vi "Resampling app.vi"() -> ()   [LabVIEW 2018]
panel:
  in  "file path (use dialog)":path
  out "error out":errorcluster
  in  "error in":errorcluster
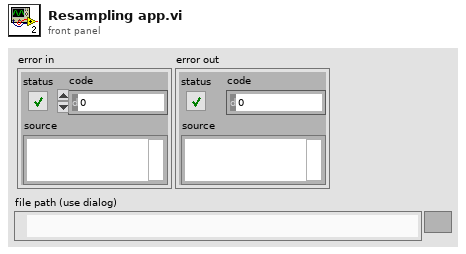
[diagram p1: front panel]
types:
  T1 = enum16{"big-endian, network order", "native, host order", "little-endian"}
  T2 = enum16{"open", "replace", "create", "open or create", "replace or create", "replace or create with confirmation"}
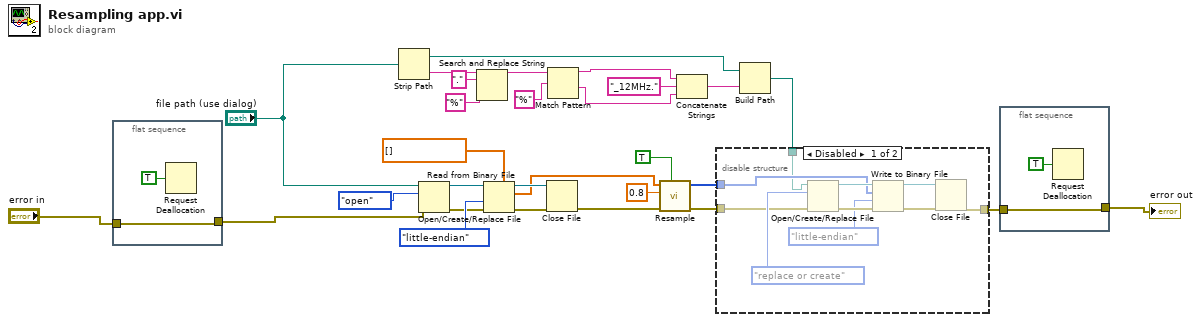
[diagram p0: block diagram]
diagram:
  n1 = flat-sequence {
    tunnel: [w30] -> w3
    tunnel: "error in" -> [w30]
    frame #0 {
      n2 = Request Deallocation(TRUE ("flag")) -> ()
    }
  }
  n3 = Strip Path(path="file path (use dialog)") -> (stripped path=w15:path, name=w10:string)
  n4 = Open/Create/Replace File(file path (use dialog)="file path (use dialog)", error in=w3, operation (0:open)=T2."open") -> (refnum out=w24:refnum<file>, error out=w26:errorcluster)  [unwired: 3 in, 1 out]
  n5 = Search and Replace String(input string=w10, search string=".", replace string="%" ("replace string (\"\")")) -> (result string=w11:string)  [unwired: 5 in, 3 out]
  n6 = Read from Binary File(5:cdb[] [], 8:w26, 9:T1."little-endian" ("byte order (0:big-endian, network order)"), 11:w24) -> (0:w25:errorcluster, 2:w22:cdb[], 3:w23:refnum<file>)  [unwired: 2 in, 1 out]
  n7 = Close File(refnum=w23, error in=w25) -> (error out=w20:errorcluster)  [unwired: 1 out]
  n8 = Match Pattern(string=w11, regular expression="%") -> (before substring=w12:string, after substring=w14:string)  [unwired: 1 in, 2 out]
  n9 = call "Resample.vi"("Resampling up"=TRUE, "error in"=w20, "New dt"=0.8, "Input data"=w22) -> ("error out"=w18:errorcluster, "IQ data"=w17:i16[])  [unwired: 6 in]
  n10 = Concatenate Strings(w12, "_12MHz." ("string"), w14) -> (w16:string)
  n11 = Build Path(base path=w15, name or relative path=w16) -> (appended path=w5:path)
  n12 = disable-structure shown="Disabled" {
    disable-tunnel: w18 -> [w35 w42]
    disable-tunnel: w17 -> [w34 _]
    disable-tunnel: w5 -> [w33 _]
    disable-tunnel: [w32 w42] -> w2
    frame Disabled {
      n13 = Open/Create/Replace File(file path (use dialog)=w33, error in=w35, operation (0:open)=T2."replace or create") -> (refnum out=w40:refnum<file>, error out=w38:errorcluster)  [unwired: 3 in, 1 out]
      n14 = Write to Binary File(file (use dialog)=w40, data=w34, error in=w38, 9:T1."little-endian" ("byte order (0:big-endian, network order)")) -> (refnum out=w41:refnum<file>, error out=w39:errorcluster)  [unwired: 2 in, 1 out]
      n15 = Close File(refnum=w41, error in=w39) -> (error out=w32:errorcluster)  [unwired: 1 out]
    }
    frame Enabled {
    }
  }
  n16 = flat-sequence {
    tunnel: [w43] -> w1
    tunnel: w2 -> [w43]
    frame #0 {
      n17 = Request Deallocation(TRUE ("flag")) -> ()
    }
  }
  "error out" <- w1
